vi "Read PWM Output Module.vi"(8 "error in":errorcluster, 11 "module in":refnum<class "Module.lvclass">) -> (0 "error out":errorcluster, 2 "channel settings":T1[](array[typedef]), 3 "module out":refnum<class "Module.lvclass">)   [LabVIEW 2020, in "Scan Engine Scripting.lvlib" / "Module.lvclass"]
uses:
  Module.lvclass
  Mode Classes/Controls/pwm channel settings.ctl
  Channel Classes/PWM Output Channel/Frequency.ctl
  Mode Classes/PWM Mode/PWM Mode.lvclass
  Channel Classes/PWM Output Channel/PWM Output Channel.lvclass
  Scan Engine Scripting.lvlib
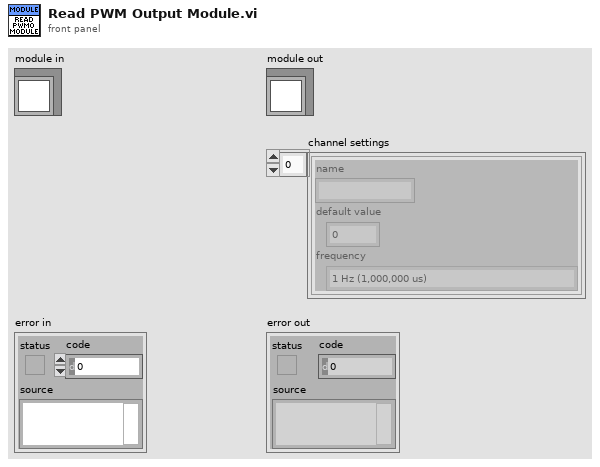
[diagram p1: front panel]
types:
  T1 = typedef "Scan Engine Scripting.lvlib/pwm channel settings.ctl" = cluster{"name":string, "default value":dbl, "frequency":T2}
  T2 = typedef "Scan Engine Scripting.lvlib/PWM Output Channel.lvclass/Frequency.ctl" = enum16{"1 Hz (1,000,000 us)", "50 Hz (20,000 us)", "250 Hz (4,000 us)", "500 Hz (2,000 us)", "1 kHz (1,000 us)", "5 kHz (200 us)", "10 kHz (100 us)", "20 kHz (50 us)"}
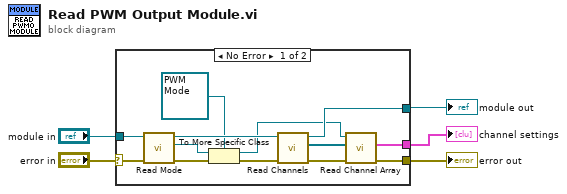
[diagram p0: block diagram]
diagram:
  n1 = case shown="No Error" "error in" {
    selector: "error in" -> [w17 w20]
    tunnel: [w7 w20] -> w2
    tunnel: [w13 w19] -> w3
    tunnel: "module in" -> [w18 w19]
    tunnel: [w6 _] -> w1
    frame No Error {
      n2 = call-dynamic "Read Mode.vi"("error in"=w17, "module in"=w18) -> ("error out"=w15:errorcluster, "mode"=w16:refnum<class "Mode.lvclass">, "module out"=w14:refnum<class "Module.lvclass">)  [unwired: 7 in]
      n3 = To More Specific Class(target class=refnum<class "PWM Mode.lvclass"> refnum ("Scan Engine Scripting.lvlib:PWM Mode.lvclass"), reference=w16, error in=w15) -> (specific class reference=w8:refnum<class "PWM Mode.lvclass">, error out=w12:errorcluster)
      n4 = call-dynamic "Read Channels.vi"("error in"=w12, "module in"=w14) -> ("error out"=w10:errorcluster, "channels"=w9:refnum<class "Channel.lvclass">[], "module out"=w13:refnum<class "Module.lvclass">)  [unwired: 7 in]
      n5 = call "Read Channel Array.vi"("error in"=w10, "channels"=w9, "PWM mode in"=w8) -> ("error out"=w7:errorcluster, "channel settings"=w6:T1[])  [unwired: 6 in, 1 out]
    }
    frame Error {
    }
  }
  "error out" <- w2
  "module out" <- w3
  "channel settings" <- w1
